vi "Correct signal gen level using PM.vi"(8 "error in (no error)":errorcluster, 9 "Power":dbl, 10 "Frequency":dbl, 11 "AM-AM in":refnum<class "AM-AM.lvclass">) -> (0 "error out":errorcluster, 2 "Power at DUT":dbl, 3 "AM-AM out":refnum<class "AM-AM.lvclass">)   [LabVIEW 2020, in "AM-AM.lvclass"]
uses:
  AM-AM.lvclass
  C:/Sandbox/Git_Sandbox/WiSpry Test Framework source code (LV20)/WiSpry Test Framework/Measurements/Measurement.lvclass
  Path Control/Paths.ctl
  AM-AM.lvclass/AM-AM.ctl
  Measurement.lvclass/Measurement.ctl
  Instruments/Signal Generator/Signal Generator.lvclass
  Instruments/Power Meter/Power Meter.lvclass
  Measurement.lvclass
  Path Control/PathControl.lvclass
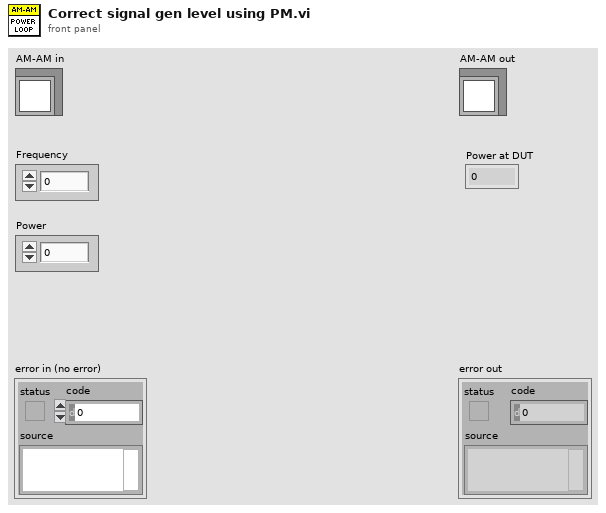
[diagram p1: front panel]
types:
  T1 = typedef "PathControl.lvclass/Paths.ctl" = enum16{"SigGen 1 -> DUT", "SigGen 2 -> DUT", "SigGen 1 -> PM 1", "SigGen 1 -> PM 2", "DUT -> SA", "DUT -> PM 2", "VSG -> DUT", "SigGen 2 -> PM 1", "SigGen 2 -> PM 2"}
  T2 = typedef "AM-AM.lvclass/Config info.ctl" = cluster{"RBW":dbl, "VBW ":dbl, "Number of Averages":dbl, "Average On":bool, "Power":cluster{"Cluster ":cluster{"From":dbl, "To":dbl, "Step":dbl}, "Array":dbl[], "Use Array":bool}, "Frequency":cluster{"Cluster ":cluster{"From":dbl, "To":dbl, "Step":dbl}, "Array":dbl[], "Use Array":bool}, "Loop order":T3, "Power Window":dbl}
  T3 = typedef "AM-AM.lvclass/Loop order.ctl" = enum16{"Device -> Power -> Frequency", "Device -> Frequency -> Power"}
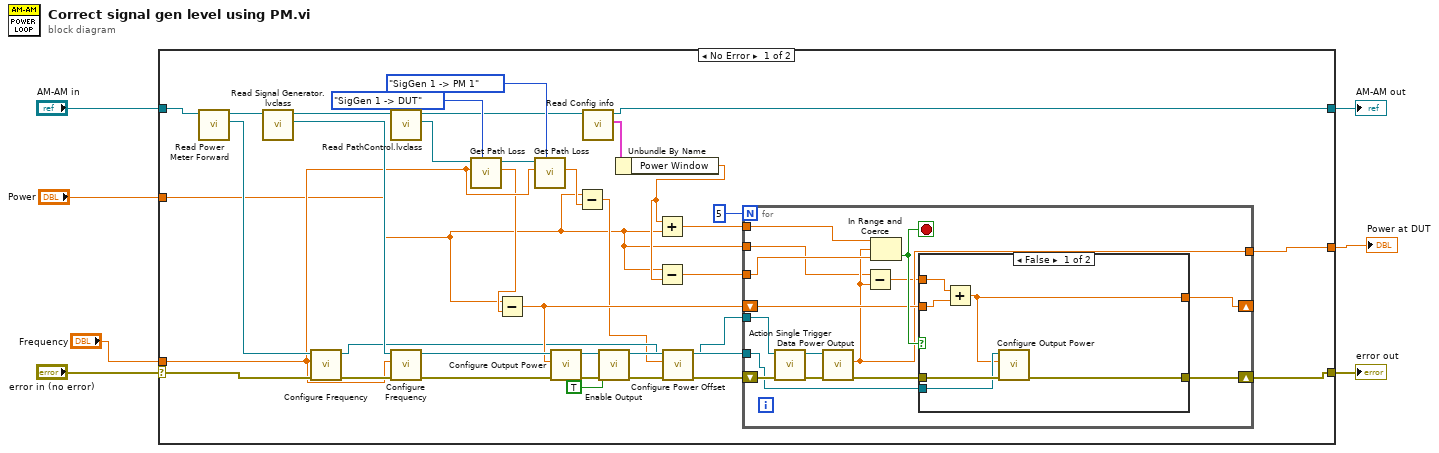
[diagram p0: block diagram]
diagram:
  n1 = case shown="No Error" "error in (no error)" {
    selector: "error in (no error)" -> [w41 w68]
    tunnel: [w17 w68] -> w6
    tunnel: [w16 w67] -> w4
    tunnel: "AM-AM in" -> [w43 w67]
    tunnel: "Frequency" -> [w32 _]
    tunnel: "Power" -> [w8 _]
    tunnel: [w9 _] -> w1
    frame No Error {
      n2 = call "Read Power Meter Forward.vi"("AM-AM in"=w43) -> ("Power Meter Forward"=w40:refnum<class "Power Meter.lvclass">, "AM-AM out"=w42:refnum<class "AM-AM.lvclass">)  [unwired: 9 in]
      n3 = call "Read Signal Generator.lvclass.vi"("AM-AM in"=w42) -> ("Signal Generator.lvclass"=w39:refnum<class "Signal Generator.lvclass">, "AM-AM out"=w37:refnum<class "AM-AM.lvclass">)  [unwired: 9 in]
      n4 = call-dynamic "Configure Frequency.vi"("error in (no error)"=w41, "Frequency"=w32, "Power Meter in"=w40) -> ("error out"=w38:errorcluster, "Power Meter out"=w13:refnum<class "Power Meter.lvclass">)  [unwired: 7 in]
      n5 = call "Read PathControl.lvclass.vi"("Measurements in"=w37) -> ("PathControl.lvclass"=w36:refnum<class "PathControl.lvclass">, "Measurements out"=w24:refnum<class "AM-AM.lvclass">)  [unwired: 9 in]
      n6 = call-dynamic "Configure Frequency.vi"("error in (no error)"=w38, "Frequency [Hz]"=w32, "Signal Generator in"=w39) -> ("error out"=w30:errorcluster, "Signal Generator out"=w29:refnum<class "Signal Generator.lvclass">)  [unwired: 7 in]
      n7 = call "Get Path Loss.vi"("Path"=Paths."SigGen 1 -> DUT", "Frequency [Hz]"=w32, "PathControl in"=w36) -> ("Insertion Loss (dB)"=w15:dbl, "PathControl out"=w34:refnum<class "PathControl.lvclass">)  [unwired: 5 in, 2 out]
      n8 = Subtract(x=w8, y=w15) -> (x-y=w18:dbl)
      n9 = call "Get Path Loss.vi"("Path"=Paths."SigGen 1 -> PM 1", "Frequency [Hz]"=w32, "PathControl in"=w34) -> ("Insertion Loss (dB)"=w31:dbl)  [unwired: 5 in, 3 out]
      n10 = call-dynamic "Configure Output Power.vi"("error in (no error)"=w30, "Output Power [dBm]"=w18, "Signal Generator in"=w29) -> ("error out"=w28:errorcluster, "Signal Generator out"=w27:refnum<class "Signal Generator.lvclass">)  [unwired: 7 in]
      n11 = Subtract(x=w8, y=w31) -> (x-y=w11:dbl)
      n12 = call "Read Config info.vi"("AM-AM in"=w24) -> ("Config info"=w23:T2, "AM-AM out"=w16:refnum<class "AM-AM.lvclass">)  [unwired: 9 in]
      n13 = call-dynamic "Enable Output.vi"("error in (no error)"=w28, "Output Enable (F)"=TRUE, "Signal Generator in"=w27) -> ("error out"=w10:errorcluster, "Signal Generator out"=w25:refnum<class "Signal Generator.lvclass">)  [unwired: 7 in]
      n14 = Unbundle By Name(w23) -> ("Power Window"=w22:dbl)
      n15 = Add(x=w22, y=w8) -> (x+y=w21:dbl)
      n16 = Subtract(x=w8, y=w22) -> (x-y=w20:dbl)
      n17 = call-dynamic "Configure Power Offset.vi"("error in (no error)"=w10, "Power Offset"=w11, "Power Meter in"=w13) -> ("error out"=w14:errorcluster, "Power Meter out"=w12:refnum<class "Power Meter.lvclass">)  [unwired: 7 in]
      n18 = for {
        N: 5 -> [_]
        shift-right: [w50] -> w17
        shift-left: w14 -> [w58]
        tunnel: w25 -> [w46]
        tunnel: w12 -> [w57]
        tunnel: w21 -> [w53]
        tunnel: w20 -> [w54]
        tunnel: [w48] -> w9
        shift-right: [w45] -> _
        shift-left: w18 -> [w49]
        tunnel: w8 -> [w44]
        stop <- w52 stop-if-true
        n19 = call-dynamic "Action Single Trigger.vi"("error in (no error)"=w58, "Power Meter in"=w57) -> ("error out"=w56:errorcluster, "Power Meter out"=w55:refnum<class "Power Meter.lvclass">)  [unwired: 8 in]
        n20 = call-dynamic "Data Power Output.vi"("error in (no error)"=w56, "Power Meter in"=w55) -> ("error out"=w51:errorcluster, "Power Out"=w48:dbl)  [unwired: 7 in, 1 out]
        n21 = Subtract(x=w44, y=w48) -> (x-y=w47:dbl)
        n22 = In Range and Coerce(upper limit=w53, x=w48, lower limit=w54) -> (In Range?=w52:bool)  [unwired: 1 out]
        n23 = case shown="False" w52 {
          tunnel: w51 -> [w62 w66]
          tunnel: [w59 w66] -> w50
          tunnel: w49 -> [w64 w65]
          tunnel: w47 -> [w63 _]
          tunnel: w46 -> [w61 _]
          tunnel: [w60 w65] -> w45
          frame False {
            n24 = Add(x=w63, y=w64) -> (x+y=w60:dbl)
            n25 = call-dynamic "Configure Output Power.vi"("error in (no error)"=w62, "Output Power [dBm]"=w60, "Signal Generator in"=w61) -> ("error out"=w59:errorcluster)  [unwired: 7 in, 1 out]
          }
          frame True {
          }
        }
      }
    }
    frame Error {
    }
  }
  "error out" <- w6
  "AM-AM out" <- w4
  "Power at DUT" <- w1
